vi "_Check_DB_Read_Length.vi"(0 "Max Size":u8=222, 1 "List of S7 Read Items":T1[](array[typedef]) {"Address Areas" items=["I/O (P)"=128, "Input (I)"=129, "Output (Q)"=130, "Bit Memory (M)"=131, "Data (DB)"=132, "Instance Data (DI)"=133, "Local Data (L)"=134, "Predecessor Local Data (VL)"=135]; "Read / Write" items=["Read"=4, "Write"=5]; "Bit Number / Byte Length" max=7 step=1}) -> (2 "Byte Length":u32, 3 "Too Long?":bool, 4 "Sorted List of S7 Read Items":T1[](array[typedef]) {"Address Areas" items=["I/O (P)"=128, "Input (I)"=129, "Output (Q)"=130, "Bit Memory (M)"=131, "Data (DB)"=132, "Instance Data (DI)"=133, "Local Data (L)"=134, "Predecessor Local Data (VL)"=135]; "Read / Write" items=["Read"=4, "Write"=5]; "Bit Number / Byte Length" max=7 step=1})   [LabVIEW 2014, in "S7 TCP.lvlib"]
uses:
  S7 TCP.lvlib
  S7 Read Write Cluster.ctl
  Data Type.ctl
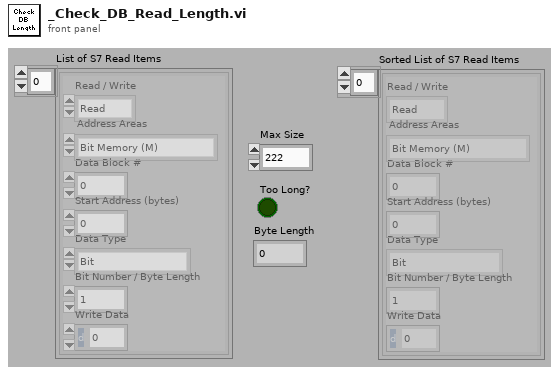
[diagram p1: front panel]
types:
  T1 = typedef "S7 TCP.lvlib/S7 Read Write Cluster.ctl" = cluster{"Read / Write":u8, "Address Areas":u8, "Data Block #":u16, "Start Address (bytes)":u32, "Data Type":T2, "Bit Number / Byte Length":u8, "Write Data":dbl}
  T2 = typedef "S7 TCP.lvlib/Data Type.ctl" = enum16{"Bit", "Byte (U8)", "Signed Byte (I8)", "Word (U16)", "Signed Word (I16)", "Long (U32)", "Signed Long (I32)", "Real (SGL)", "Defined Byte Length"}
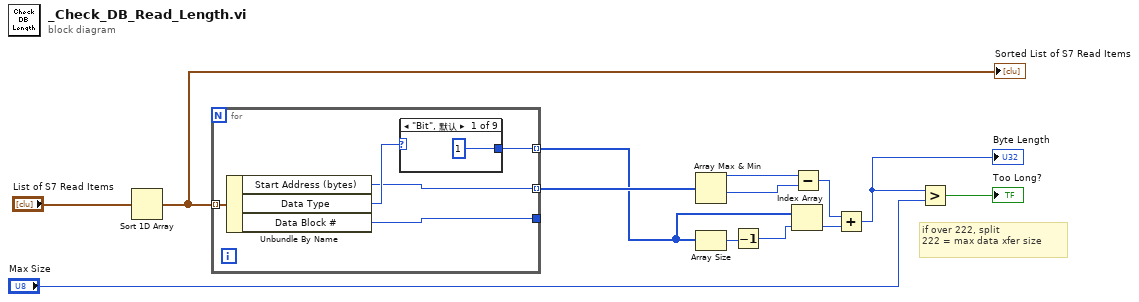
[diagram p0: block diagram]
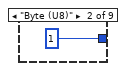
[diagram p2: hidden frame]
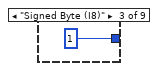
[diagram p3: hidden frame]
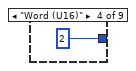
[diagram p4: hidden frame]
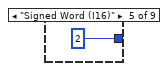
[diagram p5: hidden frame]
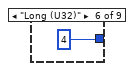
[diagram p6: hidden frame]
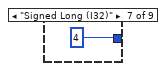
[diagram p7: hidden frame]
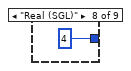
[diagram p8: hidden frame]
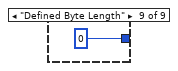
[diagram p9: hidden frame]
diagram:
  # "if over 222, split\n222 = max data xfer size"
  n1 = Sort 1D Array(array="List of S7 Read Items") -> (sorted array=w1:T1[])
  "Sorted List of S7 Read Items" <- w1
  n2 = for {
    tunnel: w1 -> [w18] mode=indexing
    tunnel: [w17] -> _
    tunnel: [w15] -> w3 mode=indexing
    tunnel: [w14] -> w2 mode=indexing
    n3 = Unbundle By Name(w18) -> ("Start Address (bytes)"=w15:u32, "Data Type"=w16:T2, "Data Block #"=w17:u16)
    n4 = case shown="\"Bit\", 默认" w16 {
      tunnel: [u8 1 ("Bit Number / Byte Length") u8 1 ("Bit Number / Byte Length") u8 1 ("Bit Number / Byte Length") u8 2 ("Bit Number / Byte Length") u8 2 ("Bit Number / Byte Length") u8 4 ("Bit Number / Byte Length") u8 4 ("Bit Number / Byte Length") u8 4 ("Bit Number / Byte Length") u8 0 ("Bit Number / Byte Length")] -> w14
      frame "Bit", Default {
      }
      frame "Byte (U8)" {
      }
      frame "Signed Byte (I8)" {
      }
      frame "Word (U16)" {
      }
      frame "Signed Word (I16)" {
      }
      frame "Long (U32)" {
      }
      frame "Signed Long (I32)" {
      }
      frame "Real (SGL)" {
      }
      frame "Defined Byte Length" {
      }
    }
  }
  n5 = Array Max & Min(array=w3) -> (max value=w5:u32, min value=w13:u32)  [unwired: 2 out]
  n6 = Array Size(array=w2) -> (size(s)=w8:i32)
  n7 = Decrement(x=w8) -> (x-1=w9:i32)
  n8 = Index Array(array=w2, index=w9) -> (element=w7:u8)
  n9 = Subtract(x=w5, y=w13) -> (x-y=w6:u32)
  n10 = Add(x=w6, y=w7) -> (x+y=w12:u32)
  "Byte Length" <- w12
  n11 = Greater?(x=w12, y="Max Size") -> (0:→"Too Long?":bool)
